vi "Configure.vi"(6 "error in":errorcluster, 8 "Configuration":T1=enum."VDC_AUTO", 9 "VISA resource name":refnum<visa-resource-name>) -> (0 "error out":errorcluster, 3 "VISA resource name out":refnum<visa-resource-name>)   [LabVIEW 2023, in "Aim TTi 1908P DMM.lvlib"]
uses:
  Aim TTi 1908P DMM.lvlib
  Configure.ctl
  5ae1b3d7-01ca-4b2a-bb66-f667e26846e6.vi
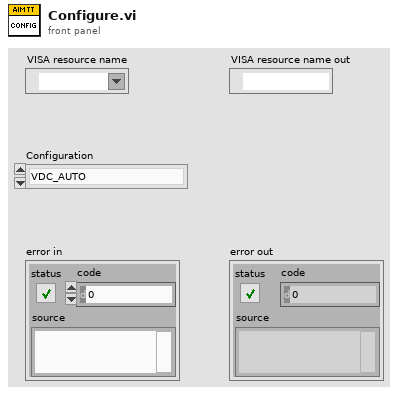
[diagram p1: front panel]
types:
  T1 = typedef "Aim TTi 1908P DMM.lvlib/Configure.ctl" = enum16{"VAC_750V", "VAC_100V", "VDC_AUTO", "VDC_100V", "VDC_1000mV", "VDC_100mV", "VDC_10V", "OHMS_AUTO", "OHMS_10K", "IDC_10A", "IDC_1mA", "IDC_100mA", "IDC_1000mA", "IAC_1mA", "IAC_100mA", "IAC_1000mA", "IAC_10A"}
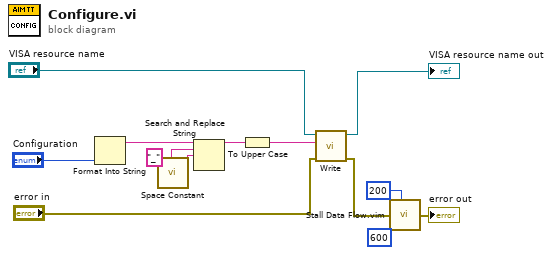
[diagram p0: block diagram]
diagram:
  (unwired) u32 600 ("milliseconds to wait")
  n1 = Format Into String("Configuration") -> (resulting string=w5:string)  [unwired: 3 in, 1 out]
  n2 = call <vilib>:"Space Constant.vi"() -> ("String"=w3:string)
  n3 = Search and Replace String(input string=w5, search string="_", replace string=w3) -> (result string=w2:string)  [unwired: 5 in, 3 out]
  n4 = To Upper Case(1:w2) -> (0:w1:string)
  n5 = call "Write.vi"("error in"="error in", "Data to write"=w1, "VISA resource name"="VISA resource name") -> ("error out"=w9:errorcluster, "VISA resource name out"=→"VISA resource name out":refnum<visa-resource-name>)  [unwired: 5 in]
  n6 = call "Stall Data Flow.vim"("value in"=w9, "milliseconds to wait"=u32 200) -> ("value out"=→"error out":errorcluster)  [unwired: 1 out]
